vi "AnalogSignalToByte.vi"(2 "Offset":dbl format="%#_16g", 3 "Resolution":dbl format="%#_16g", 4 "Value":dbl format="%#_16g") -> (0 "HighByte":u8, 1 "LowByte":u8)   [LabVIEW 2013]
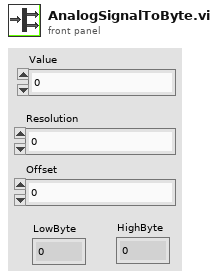
[diagram p1: front panel]
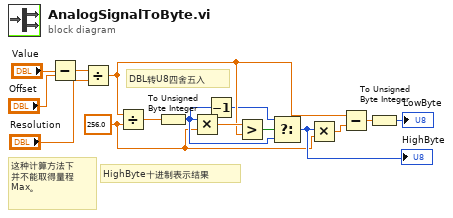
[diagram p0: block diagram]
diagram:
  w1 = 256.0 ("y")
  # "DBL转U8四舍五入"
  # "HighByte十进制表示结果"
  # "这种计算方法下\n并不能取得量程\nMax。"
  n1 = Subtract(x="Value", y="Offset") -> (x-y=w6:dbl)
  n2 = Divide(x=w6, y="Resolution") -> (x/y=w9:dbl)
  n3 = Divide(x=w9, y=w1) -> (x/y=w12:dbl)
  n4 = To Unsigned Byte Integer(number=w12) -> (unsigned 8bit integer=w3:u8)
  n5 = Multiply(x=w3, y=w1) -> (x*y=w11:dbl)
  n6 = Decrement(x=w3) -> (x-1=w4:u8)
  n7 = Greater?(x=w11, y=w9) -> (0:w5:bool)
  n8 = Select(t=w4, s=w5, f=w3) -> (s? t:f=w2:u8)
  "HighByte" <- w2
  n9 = Multiply(x=w2, y=w1) -> (x*y=w10:dbl)
  n10 = Subtract(x=w9, y=w10) -> (x-y=w8:dbl)
  n11 = To Unsigned Byte Integer(number=w8) -> (unsigned 8bit integer=→"LowByte":u8)
